vi "Metal_alpha.vi"(1 "Metal_Type":string) -> (0 "alpha (/K)":dbl)   [LabVIEW 2011]
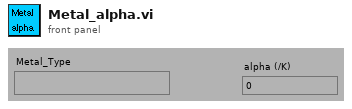
[diagram p1: front panel]
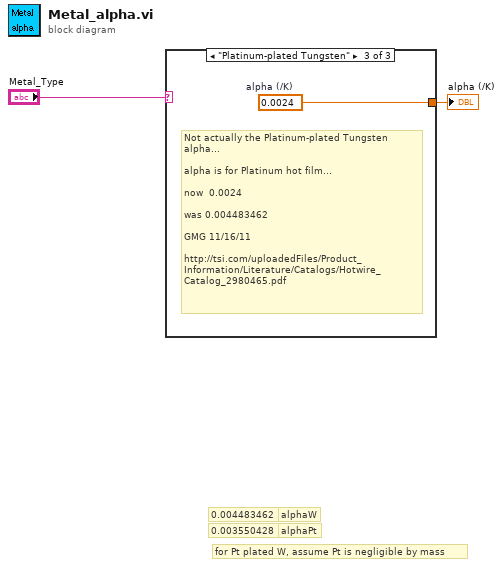
[diagram p0: block diagram]
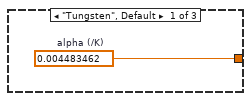
[diagram p2: hidden frame]
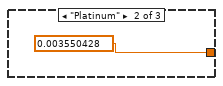
[diagram p3: hidden frame]
diagram:
  # "for Pt plated W, assume Pt is negligible by mass"
  # "alphaPt"
  # "alphaW"
  # "0.003550428"
  # "0.004483462"
  n1 = case shown="\"Platinum-plated Tungsten\"" "Metal_Type" {
    tunnel: [w3 0.003550428 w5] -> w1
    frame "Tungsten", Default {
      w3 = 0.004483462  # alpha (/K)
    }
    frame "Platinum" {
    }
    frame "Platinum-plated Tungsten" {
      w5 = 0.0024  # alpha (/K)
      # "Not actually the Platinum-plated Tungsten\nalpha...\n\nalpha is for Platinum hot film...\n\nnow  0.0024\n\nwas 0.004483462 \n\nGMG 11/16/11\n\nhttp://tsi.com/uploadedFiles/Product_Information/Literature/Catalogs/Hotwire_Catalog_2980465.pdf"
    }
  }
  "alpha (/K)" <- w1
